vi "數位積分版(無數位濾波)V5.vi"() -> ()   [LabVIEW 2010]
uses:
  <vilib>/DAQmx/read.llb/DAQmx Read (Analog DBL 1Chan 1Samp).vi
  <vilib>/DAQmx/write.llb/DAQmx Write (Analog DBL 1Chan 1Samp).vi
  <vilib>/DAQmx/create/channels.llb/DAQmx Create Channel (AI-Voltage-Basic).vi
  <vilib>/DAQmx/configure/timing.llb/DAQmx Timing (Sample Clock).vi
  <vilib>/DAQmx/create/channels.llb/DAQmx Create Channel (AO-Voltage-Basic).vi
  <vilib>/daqmx/miscellaneous.llb/DAQmx Fill In Error Info.vi
panel:
  out "Waveform Chart":dbl(graph)
  in  "輸入訊號縮放比例":dbl=1.0
  in  "ÂoDC?":bool
  in  "Kv":dbl=-5000.0
  in  "濾波?":bool
  out "理想迴圈時間":dbl
  out "延遲警告":bool
  out "當下DC值":dbl
  in  "DAQ input":tag
  in  "DAQ output":tag
  in  "Ka":dbl=-300.0
  out "message":string=" INSTRUCTIONS:\r\rNormal Use:  When using subVIs that incorporate the error in/error out (or error I/O) structure, place this handler where you want to inform the user of an error, typically at the end of the I/O data path, as the last action of the program.  If the error in error? is ERROR, the handler creates a message describing the error and its source.  If the type of dialog = 1 (default), the message is displayed to the user, who can only acknowedge it.  If the type = 2, the user can acknowledge the message or abort execution; aborting a program with active I/O is not recommended.  If the type = 0, no message is displayed; this is used to process the error programmatically, and the error out cluster elements are wired to individual terminals for that reason.  \r\rOther Use:\n\r\nlocal testing.  To test the error code of a subVI or function that does not have the error I/O structure, you can wire its error code and a source string to the local error code and error source inputs.  If error in error? indicates no error and error code is not equal to 0, the local code and source are substituted for the error in values, and error? is set TRUE (ERROR)."
  out "while平均運行時間":dbl
  in  "取樣頻率":dbl=5000.0 min=1.0 max=20000.0 step=1.0
  in  "stop":bool
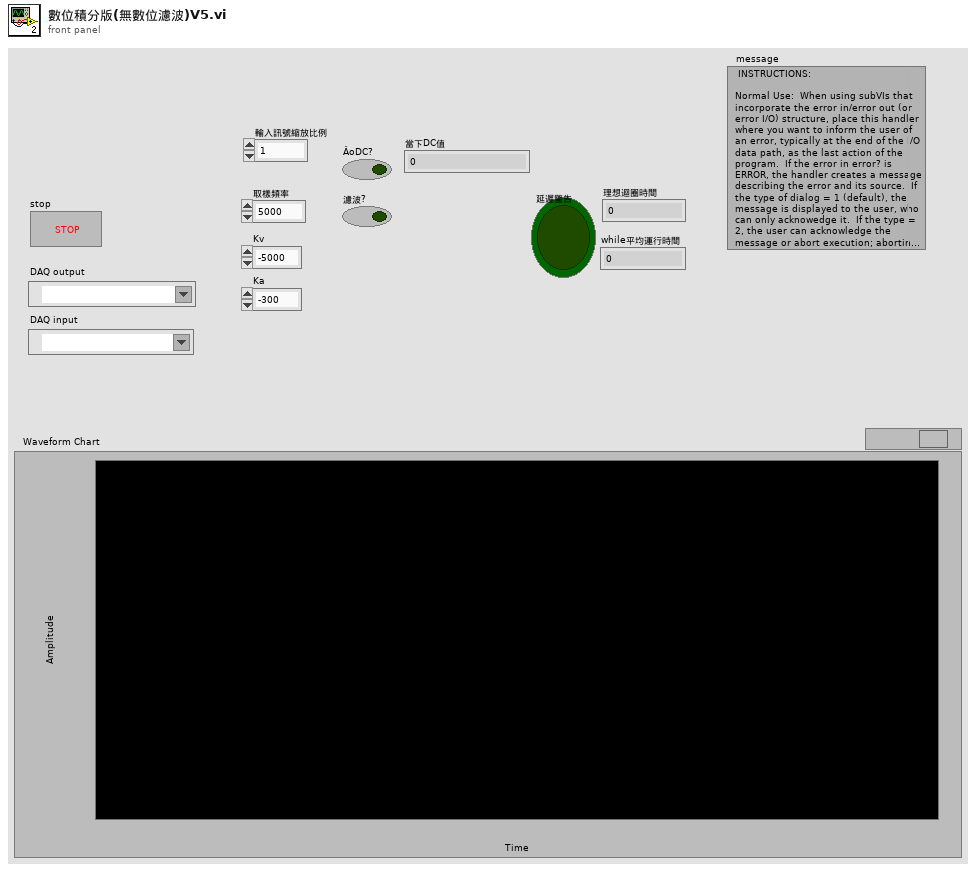
[diagram p1: front panel]
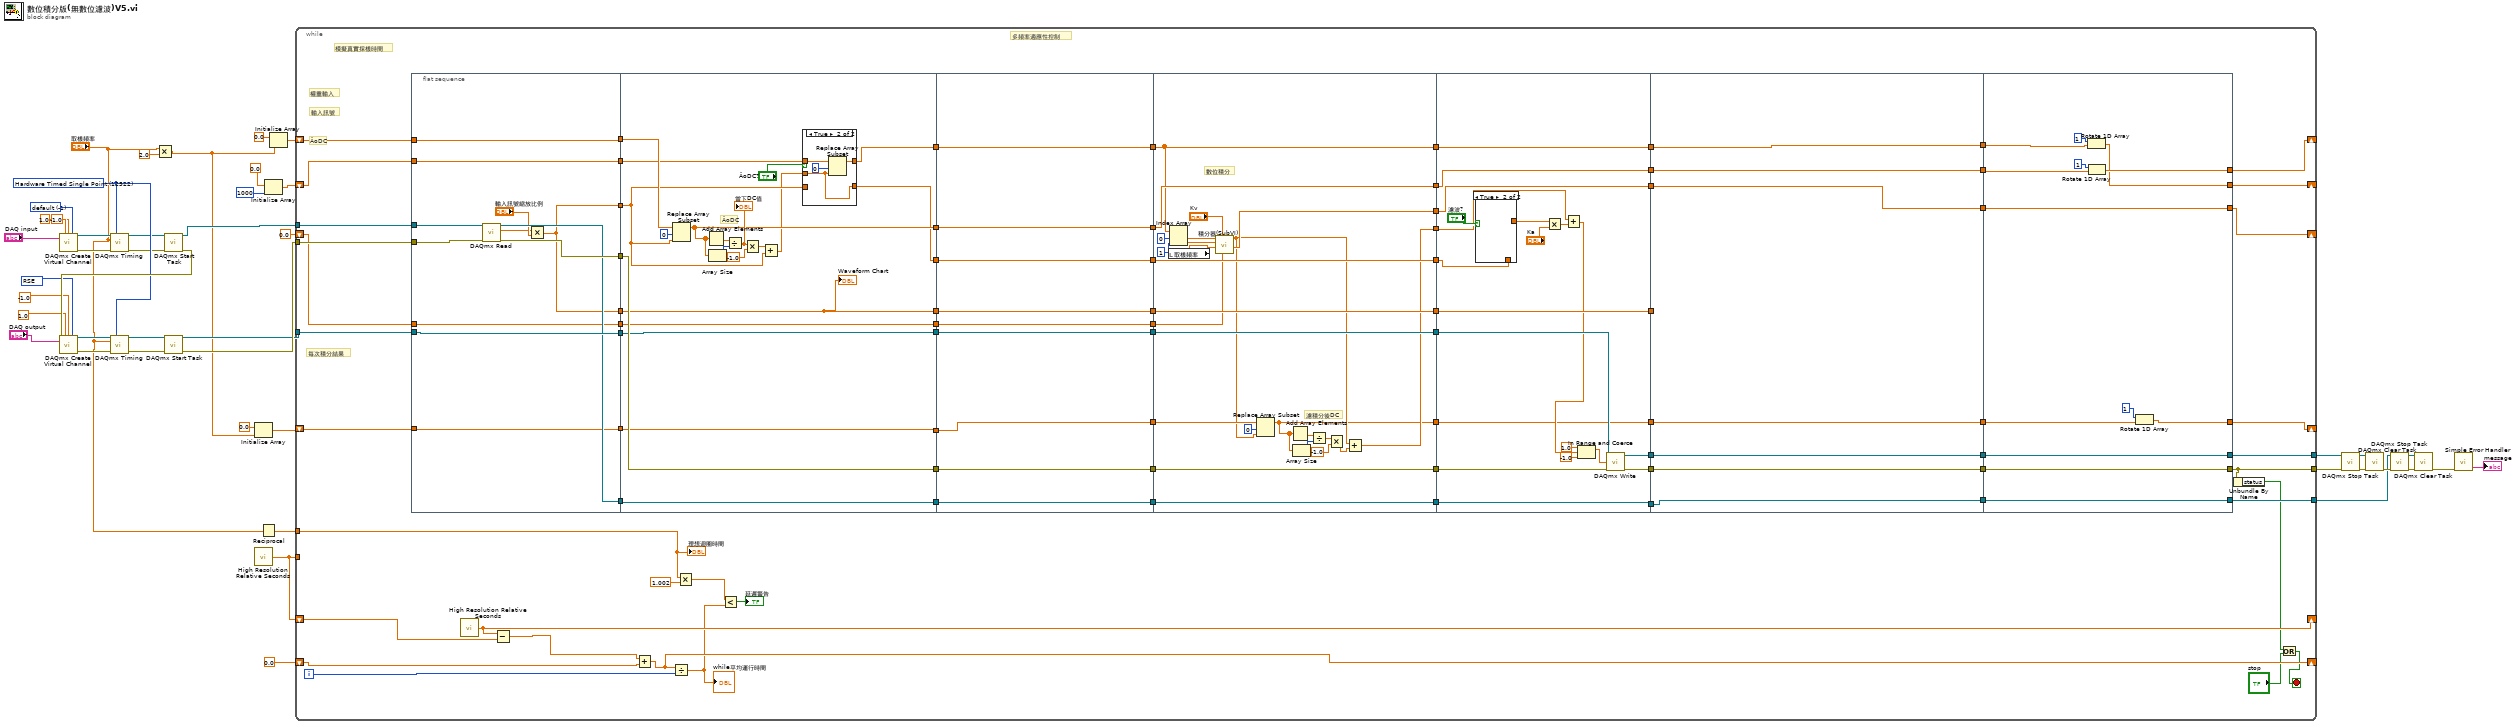
[diagram p0: block diagram]
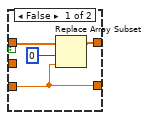
[diagram p2: hidden frame]
diagram:
  w39 = 12522 items=["Finite Samples"=10178, "Continuous Samples"=10123, "Hardware Timed Single Point"=12522] ("sample mode")
  w36 = 10083 items=["Default"=-1, "RSE"=10083, "Differential"=10106, "Pseudodifferential"=12529] ("output terminal configuration")
  w35 = -1 items=["default"=-1, "RSE"=10083, "NRSE"=10078, "Differential"=10106, "Pseudodifferential"=12529] ("input terminal configuration")
  n1 = call-poly <vilib>:"DAQmx Create Virtual Channel.vi"("maximum value"=1.0, "minimum value"=-1.0, "input terminal configuration"=w35, "physical channels"="DAQ input") -> ("task out"=w27:refnum<k21>, "error out"=w30:errorcluster)  [unwired: 10 in]
  n2 = call-poly <vilib>:"DAQmx Timing.vi"("task/channels in"=w27, "sample mode"=w39, "rate"="取樣頻率", "error in"=w30) -> ("task out"=w28:refnum<k21>, "error out"=w29:errorcluster)  [unwired: 10 in]
  n3 = Multiply(x="取樣頻率", y=2.0) -> (x*y=w1:dbl)
  n4 = call <vilib>:"DAQmx Start Task.vi"("task/channels in"=w28, "error in"=w29) -> ("task out"=w7:refnum<k21>, "error out"=w42:errorcluster)  [unwired: 12 in]
  n5 = call-poly <vilib>:"DAQmx Create Virtual Channel.vi"("maximum value"=1.0, "minimum value"=-1.0, "output terminal configuration"=w36, "physical channels"="DAQ output", "error in"=w42) -> ("task out"=w34:refnum<k21>, "error out"=w31:errorcluster)  [unwired: 9 in]
  n6 = call-poly <vilib>:"DAQmx Timing.vi"("task/channels in"=w34, "sample mode"=w39, "rate"="取樣頻率", "error in"=w31) -> ("task out"=w33:refnum<k21>, "error out"=w32:errorcluster)  [unwired: 10 in]
  n7 = call <vilib>:"DAQmx Start Task.vi"("task/channels in"=w33, "error in"=w32) -> ("task out"=w25:refnum<k21>, "error out"=w26:errorcluster)  [unwired: 12 in]
  n8 = Initialize Array(0.0 ("element"), w1) -> (w5:dbl[])
  n9 = call <vilib>:"High Resolution Relative Seconds.vi"() -> ("relative seconds"=w45:dbl)
  n10 = Reciprocal(x="取樣頻率") -> (1/x=w10:dbl)
  n11 = Initialize Array(0.0 ("element"), 1000 ("dimension size")) -> (w11:dbl[])
  n12 = Initialize Array(0.0 ("element"), w1) -> (w13:dbl[])
  n13 = while {
    tunnel: w45 -> [_]
    shift-right: [w121] -> _
    shift-left: w45 -> [w120]
    shift-right: [w122] -> _
    shift-left: 0.0 -> [w124]
    shift-right: [w114] -> _
    shift-left: w13 -> [w116]
    tunnel: w7 -> [w111]
    tunnel: w26 -> [w110]
    tunnel: w25 -> [w109]
    tunnel: [w105] -> w19
    tunnel: [w96] -> w18
    tunnel: [w99] -> w17
    shift-right: [w83] -> _
    shift-left: w11 -> [w87]
    tunnel: w10 -> [w81]
    shift-right: [w71] -> _
    shift-left: 0.0 ("輸出累加ERR回朔") -> [w76]
    shift-right: [w49] -> _
    shift-left: w5 -> [w53]
    i -> [w123]
    stop <- w98 stop-if-true
    # "每次積分結果"
    # "權重輸入"
    # "輸入訊號"
    # "ÂoDC"
    # "模擬真實採樣時間"
    # "多頻率適應性控制"
    n14 = flat-sequence {
      tunnel: [w127] -> w125
      tunnel: [w127] -> w118
      tunnel: [w134] -> w117
      tunnel: w116 -> [w137]
      tunnel: [w137] -> w115
      tunnel: w111 -> [w136]
      tunnel: w110 -> [w135]
      tunnel: w109 -> [w133]
      tunnel: [w133] -> w108
      tunnel: [w132] -> w102
      tunnel: [w131] -> w88
      tunnel: w87 -> [w131]
      tunnel: w76 -> [w130]
      tunnel: [w130] -> w75
      tunnel: [w129] -> w54
      tunnel: w53 -> [w129]
      tunnel: w125 -> [w141]
      tunnel: [w157] -> w70
      tunnel: [w138] -> w68
      tunnel: w118 -> [w138]
      tunnel: w117 -> [w157]
      tunnel: w115 -> [w155]
      tunnel: [w142] -> w66
      tunnel: [w149] -> w64
      tunnel: w108 -> [w149]
      tunnel: [w148] -> w62
      tunnel: w102 -> [w148]
      tunnel: w88 -> [w147]
      tunnel: [w146] -> w60
      tunnel: w75 -> [w144]
      tunnel: [w145] -> w58
      tunnel: [w144] -> w56
      tunnel: w54 -> [w140]
      tunnel: [w140] -> w52
      tunnel: w70 -> [w174]
      tunnel: [w174] -> w69
      tunnel: w68 -> [w173]
      tunnel: [w173] -> w67
      tunnel: w66 -> [w172]
      tunnel: [w172] -> w65
      tunnel: w64 -> [w171]
      tunnel: [w171] -> w63
      tunnel: w62 -> [w170]
      tunnel: [w170] -> w61
      tunnel: w60 -> [w167]
      tunnel: [w167] -> w59
      tunnel: w58 -> [w169]
      tunnel: [w169] -> w57
      tunnel: w56 -> [w168]
      tunnel: [w168] -> w55
      tunnel: w52 -> [w166]
      tunnel: [w166] -> w51
      tunnel: w69 -> [w199]
      tunnel: [w199] -> w94
      tunnel: w67 -> [w198]
      tunnel: [w198] -> w93
      tunnel: [w189] -> w92
      tunnel: w65 -> [w197]
      tunnel: [w197] -> w91
      tunnel: w63 -> [w196]
      tunnel: [w196] -> w90
      tunnel: w61 -> [w195]
      tunnel: [w195] -> w89
      tunnel: [w186] -> w84
      tunnel: w59 -> [w186]
      tunnel: w57 -> [w189]
      tunnel: [w185] -> w73
      tunnel: w55 -> [w190]
      tunnel: w51 -> [w179]
      tunnel: [w176] -> w50
      tunnel: [w175] -> w46
      tunnel: w94 -> [w216]
      tunnel: [w208] -> w119
      tunnel: w93 -> [w208]
      tunnel: [w218] -> w112
      tunnel: w92 -> [w218]
      tunnel: w91 -> [w205]
      tunnel: w90 -> [w217]
      tunnel: [w215] -> w106
      tunnel: [w214] -> w104
      tunnel: w89 -> [w213]
      tunnel: [w213] -> w101
      tunnel: [w209] -> w85
      tunnel: w84 -> [w209]
      tunnel: [w204] -> w74
      tunnel: w73 -> [w204]
      tunnel: w50 -> [w202]
      tunnel: [w200] -> w47
      tunnel: w46 -> [w200]
      tunnel: w119 -> [_]
      tunnel: [w224] -> w113
      tunnel: w112 -> [w224]
      tunnel: [w227] -> w107
      tunnel: w106 -> [w227]
      tunnel: w104 -> [w226]
      tunnel: [w226] -> w103
      tunnel: w101 -> [w225]
      tunnel: [w225] -> w100
      tunnel: [w223] -> w86
      tunnel: w85 -> [w223]
      tunnel: w74 -> [w222]
      tunnel: [w222] -> w72
      tunnel: [w221] -> w48
      tunnel: w47 -> [w221]
      tunnel: [w239] -> w114
      tunnel: w113 -> [w238]
      tunnel: w107 -> [w237]
      tunnel: [w237] -> w105
      tunnel: [w236] -> w96
      tunnel: w103 -> [w236]
      tunnel: w100 -> [w235]
      tunnel: [w235] -> w99
      tunnel: w86 -> [w233]
      tunnel: [w232] -> w83
      tunnel: [w231] -> w71
      tunnel: w72 -> [w231]
      tunnel: [w228] -> w49
      tunnel: w48 -> [w229]
      frame #0 {
        n15 = call-poly <vilib>:"DAQmx Read.vi"("task/channels in"=w136, "error in"=w135) -> ("task out"=w132:refnum<k21>, "data"=w126:dbl, "error out"=w134:errorcluster)  [unwired: 11 in]
        n16 = Multiply(x=w126, y="輸入訊號縮放比例") -> (x*y=w127:dbl)
      }
      frame #1 {
        # "ÂoDC"
        n17 = Replace Array Subset(array=w155, new element=w141, index=0) -> (w145:dbl[])
        n18 = Add Array Elements(numeric array=w145) -> (sum=w154:dbl)
        n19 = Array Size(array=w145) -> (size(s)=w153:i32)
        n20 = Divide(x=w154, y=w153) -> (x/y=w152:dbl)
        "當下DC值" <- w152
        n21 = Multiply(x=w152, y=-1.0) -> (x*y=w150:dbl)
        n22 = Add(x=w150, y=w141) -> (x+y=w139:dbl)
        n23 = case shown="True" "ÂoDC?" {
          tunnel: w147 -> [w159 w164]
          tunnel: [w160 w163] -> w146
          tunnel: w139 -> [_ w162]
          tunnel: w141 -> [w158 _]
          tunnel: [w158 w162] -> w142
          frame False {
            n24 = Replace Array Subset(array=w159, new element=w158, index=0) -> (w160:dbl[])
          }
          frame True {
            n25 = Replace Array Subset(array=w164, new element=w162, index=0) -> (w163:dbl[])
          }
        }
        "Waveform Chart" <- w138
      }
      frame #2 {
      }
      frame #3 {
        # "濾積分後DC"
        # "數位積分"
        n26 = local read "取樣頻率"() -> (w188:dbl)
        n27 = Index Array(array=w186, index #1=0 ("index"), index #2=1 ("index")) -> (element #1=w192:dbl, element #2=w191:dbl)
        n28 = call "積分器(SubVI).vi"("輸入累加ERR回朔"=w190, "I增益"="Kv", "samples (Hz)"=w188, "前一個ERR"=w191, "當下ERR"=w192) -> ("輸出累加ERR回朔"=w185:dbl, "積分修正量"=w178:dbl)  [unwired: 5 in]
        n29 = Replace Array Subset(array=w179, new element=w178, index=0) -> (w175:dbl[])
        n30 = Add Array Elements(numeric array=w175) -> (sum=w183:dbl)
        n31 = Array Size(array=w175) -> (size(s)=w182:i32)
        n32 = Divide(x=w183, y=w182) -> (x/y=w181:dbl)
        n33 = Multiply(x=w181, y=-1.0) -> (x*y=w177:dbl)
        n34 = Add(x=w178, y=w177) -> (x+y=w176:dbl)
      }
      frame #4 {
        n35 = case shown="True" "濾波?" {
          tunnel: [w220 _] -> w206
          tunnel: w205 -> [w220 _]
          frame False {
          }
          frame True {
          }
        }
        n36 = Multiply(x=w206, y="Ka") -> (x*y=w203:dbl)
        n37 = Add(x=w202, y=w203) -> (x+y=w201:dbl)
        n38 = In Range and Coerce(upper limit=1.0, x=w201, lower limit=-1.0) -> (coerced(x)=w212:dbl)  [unwired: 1 out]
        n39 = call-poly <vilib>:"DAQmx Write.vi"("task/channels in"=w217, "data"=w212, "error in"=w216) -> ("task out"=w215:refnum<k21>, "error out"=w214:errorcluster)  [unwired: 10 in, 1 out]
      }
      frame #5 {
      }
      frame #6 {
        n40 = Rotate 1D Array(1:w233, 2:1 ("n")) -> (0:w232:dbl[])
        n41 = Rotate 1D Array(1:w238, 2:1 ("n")) -> (0:w239:dbl[])
        n42 = Rotate 1D Array(1:w229, 2:1 ("n")) -> (0:w228:dbl[])
      }
    }
    n43 = call <vilib>:"High Resolution Relative Seconds.vi"() -> ("relative seconds"=w121:dbl)
    n44 = Subtract(x=w121, y=w120) -> (x-y=w82:dbl)
    n45 = Add(x=w82, y=w124) -> (x+y=w122:dbl)
    n46 = Divide(x=w122, y=w123) -> (x/y=w78:dbl)
    "while平均運行時間" <- w78
    n47 = Multiply(x=w81, y=1.002) -> (x*y=w79:dbl)
    n48 = Less?(x=w79, y=w78) -> (x < y?=→"延遲警告":bool)
    n49 = Unbundle By Name(w96) -> ("status"=w95:bool)
    n50 = Or(x=w95, y="stop") -> (x .or. y?=w98:bool)
    "理想迴圈時間" <- w81
  }
  n51 = call <vilib>:"DAQmx Stop Task.vi"("task/channels in"=w19, "error in"=w18) -> ("task out"=w20:refnum<k21>, "error out"=w21:errorcluster)  [unwired: 12 in]
  n52 = call <vilib>:"DAQmx Clear Task.vi"("task in"=w20, "error in"=w21) -> ("error out"=w24:errorcluster)  [unwired: 13 in]
  n53 = call <vilib>:"DAQmx Stop Task.vi"("task/channels in"=w17, "error in"=w24) -> ("task out"=w23:refnum<k21>, "error out"=w22:errorcluster)  [unwired: 12 in]
  n54 = call <vilib>:"DAQmx Clear Task.vi"("task in"=w23, "error in"=w22) -> ("error out"=w16:errorcluster)  [unwired: 13 in]
  n55 = call <vilib>:"Simple Error Handler.vi"("error in (no error)"=w16) -> ("message"=→"message":string)  [unwired: 4 in, 4 out]
